vi "ConvertGoop2ToGoop3_GetGoop2ClassInheritance.vi"(0 "application reference (local)":refnum<vi>, 1 "Goop2VIPath(has to use GOOPKernel)":path, 5 "error in (no error)":errorcluster) -> (15 "Inheritance":path[](array[path]), 19 "error out":errorcluster)   [LabVIEW 2020]
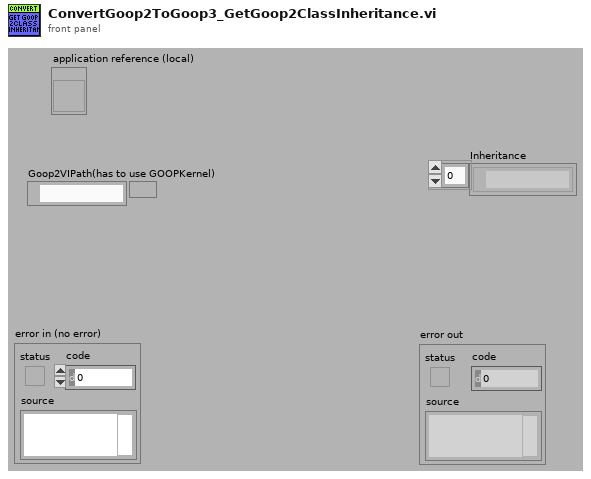
[diagram p1: front panel]
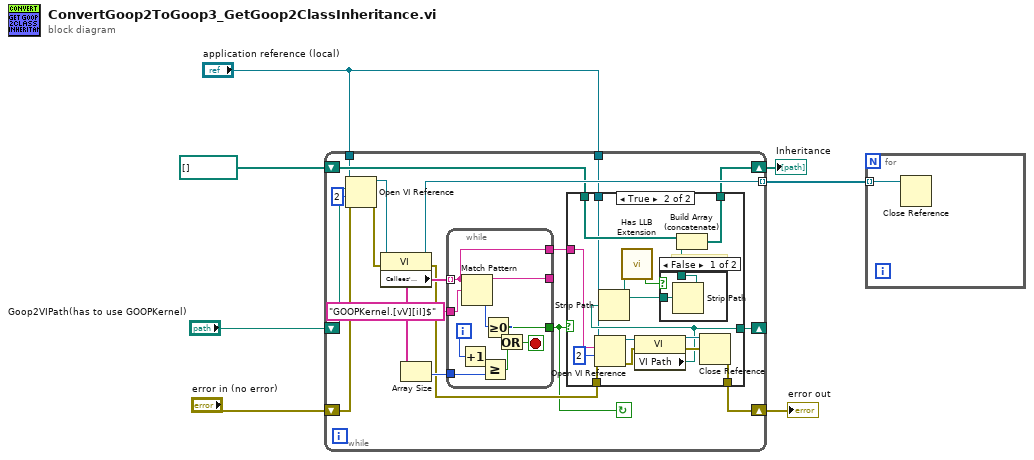
[diagram p0: block diagram]
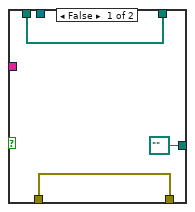
[diagram p2: hidden frame]
diagram:
  n1 = while {
    shift-right: [w16] -> w5
    shift-left: "error in (no error)" -> [w18]
    tunnel: [w15] -> w2 mode=indexing
    shift-right: [w14] -> _
    shift-left: "Goop2VIPath(has to use GOOPKernel)" -> [w11]
    shift-right: [w12] -> w3
    shift-left: path[] [] -> [w13]
    tunnel: "application reference (local)" -> [w10]
    tunnel: "application reference (local)" -> [w9]
    stop <- w17 continue-if-true
    n2 = Open VI Reference(application reference (local)=w9, vi path=w11, options=2, error in (no error)=w18) -> (vi reference=w25:refnum<vi>, error out=w24:errorcluster)  [unwired: 2 in]
    n3 = property class="VI"(reference=w25, error in=w24) -> (reference out=w15:refnum<vi>, error out=w19:errorcluster, "Callees' Names"=w23:string[])
    n4 = Array Size(array=w23) -> (size(s)=w21:i32)
    n5 = while {
      tunnel: w23 -> [w49] mode=indexing
      tunnel: "GOOPKernel.[vV][iI]$" ("string") -> [w56]
      tunnel: w21 -> [w47]
      tunnel: [w51] -> w17
      tunnel: [w50] -> _
      tunnel: [w49] -> w20
      i -> [w55]
      stop <- w52 stop-if-true
      n6 = Increment(x=w55) -> (x+1=w48:i32)
      n7 = Match Pattern(string=w49, regular expression=w56) -> (before substring=w50:string, offset past match=w54:i32)  [unwired: 1 in, 2 out]
      n8 = Greater Or Equal?(x=w48, y=w47) -> (x >= y?=w53:bool)
      n9 = Greater Or Equal To 0?(x=w54) -> (x >= 0?=w51:bool)
      n10 = Or(x=w51, y=w53) -> (x .or. y?=w52:bool)
    }
    n11 = case shown="True" w17 {
      tunnel: w20 -> [_ w43]
      tunnel: w19 -> [w28 w38]
      tunnel: [w28 w37] -> w16
      tunnel: w13 -> [w27 w34]
      tunnel: [w27 w33] -> w12
      tunnel: [path "" ("Path") w36] -> w14
      tunnel: w10 -> [_ w30]
      frame False {
      }
      frame True {
        # "Iheritance"
        n12 = Open VI Reference(application reference (local)=w30, vi path=w43, options=2, error in (no error)=w38) -> (vi reference=w42:refnum<vi>, error out=w41:errorcluster)  [unwired: 2 in]
        n13 = property class="VI"(reference=w42, error in=w41) -> (reference out=w40:refnum<vi>, error out=w39:errorcluster, "VI Path"=w36:path)
        n14 = Strip Path(path=w36) -> (stripped path=w31:path)  [unwired: 1 out]
        n15 = call <vilib>:"Has LLB Extension.vi"("path"=w31) -> ("path to VI library?"=w32:bool)
        n16 = case shown="False" w32 {
          tunnel: [w44 w46] -> w35
          tunnel: w31 -> [w45 w46]
          frame False {
            n17 = Strip Path(path=w45) -> (stripped path=w44:path)  [unwired: 1 out]
          }
          frame True {
          }
        }
        n18 = Build Array (concatenate)(w34, w35) -> (w33:path[])
        n19 = Close Reference(reference=w40, error in (no error)=w39) -> (error out=w37:errorcluster)
      }
    }
  }
  "error out" <- w5
  "Inheritance" <- w3
  n20 = for {
    tunnel: w2 -> [w57] mode=indexing
    n21 = Close Reference(reference=w57) -> ()  [unwired: 1 in, 1 out]
  }
